vi "Begin.vi"() -> (0 "error out":errorcluster, 1 "CameraDevRef":T5)   [LabVIEW 2011]
doc: "Called before other user functions, this VI is expected to open initial I/O refnums, load in file data, and do all program initialization. Notice that the <B>error out</B> terminal is simply used for data flow. Wiring it to other structures or subVIs ensures that this VI runs first."
uses:
  <vilib>/Rock Robotics/WPI/Camera/WPI_CameraDevRef.ctl
  <vilib>/Rock Robotics/WPI/Encoder/WPI_EncoderDevRef.ctl
  <vilib>/Rock Robotics/SystemInterfaces/Encoder/FPGA_EncoderIdx.ctl
  <vilib>/Rock Robotics/SystemInterfaces/Counter/FPGA_CounterCtrSystemIndex.ctl
  <vilib>/Rock Robotics/WPI/Encoder/WPI_EncoderType.ctl
  <vilib>/Rock Robotics/SystemInterfaces/DIO/FPGA_DIOPWMChannel.ctl
  <vilib>/Rock Robotics/WPI/Joystick/WPI_JoystickDeviceEnum.ctl
  <vilib>/Rock Robotics/WPI/Relay/WPI_RelayDirection.ctl
  <vilib>/Rock Robotics/SystemInterfaces/DIO/FPGA_DIORelayChannel.ctl
  <vilib>/Rock Robotics/SystemInterfaces/Typedef/FPGA_TypedefDigitalModule.ctl
  <vilib>/Rock Robotics/SystemInterfaces/AI/FPGA_AIChannel.ctl
  <vilib>/Rock Robotics/SystemInterfaces/AI/FPGA_AIGyroChannel.ctl
  <vilib>/Rock Robotics/SystemInterfaces/DIO/FPGA_DIOChannel.ctl
  <vilib>/Rock Robotics/WPI/MotorControl/WPI_MotorControlOpen Jaguar.vi
  <vilib>/Rock Robotics/WPI/MotorControl/WPI_MotorControlOpen Victor.vi
  Robot Global Data.vi
  <vilib>/Rock Robotics/WPI/Counter/WPI_CounterDigitalInputToDigitalSource.vi
panel:
  out "EncoderDevRef 2":T1={"DevStatus"={"status"=FALSE, "code"=0, "source"=""}, "EncoderIndex"=enum."Invalid", "CounterIndex"=enum."Invalid", "DistancePerCount"=1.0, "Decoding Type"=enum."4x"}
  out "LDriveEncoder 2":errorcluster
  out "EncoderDevRef":T1={"DevStatus"={"status"=FALSE, "code"=0, "source"=""}, "EncoderIndex"=enum."Invalid", "CounterIndex"=enum."Invalid", "DistancePerCount"=1.0, "Decoding Type"=enum."4x"}
  out "LDriveEncoder":errorcluster
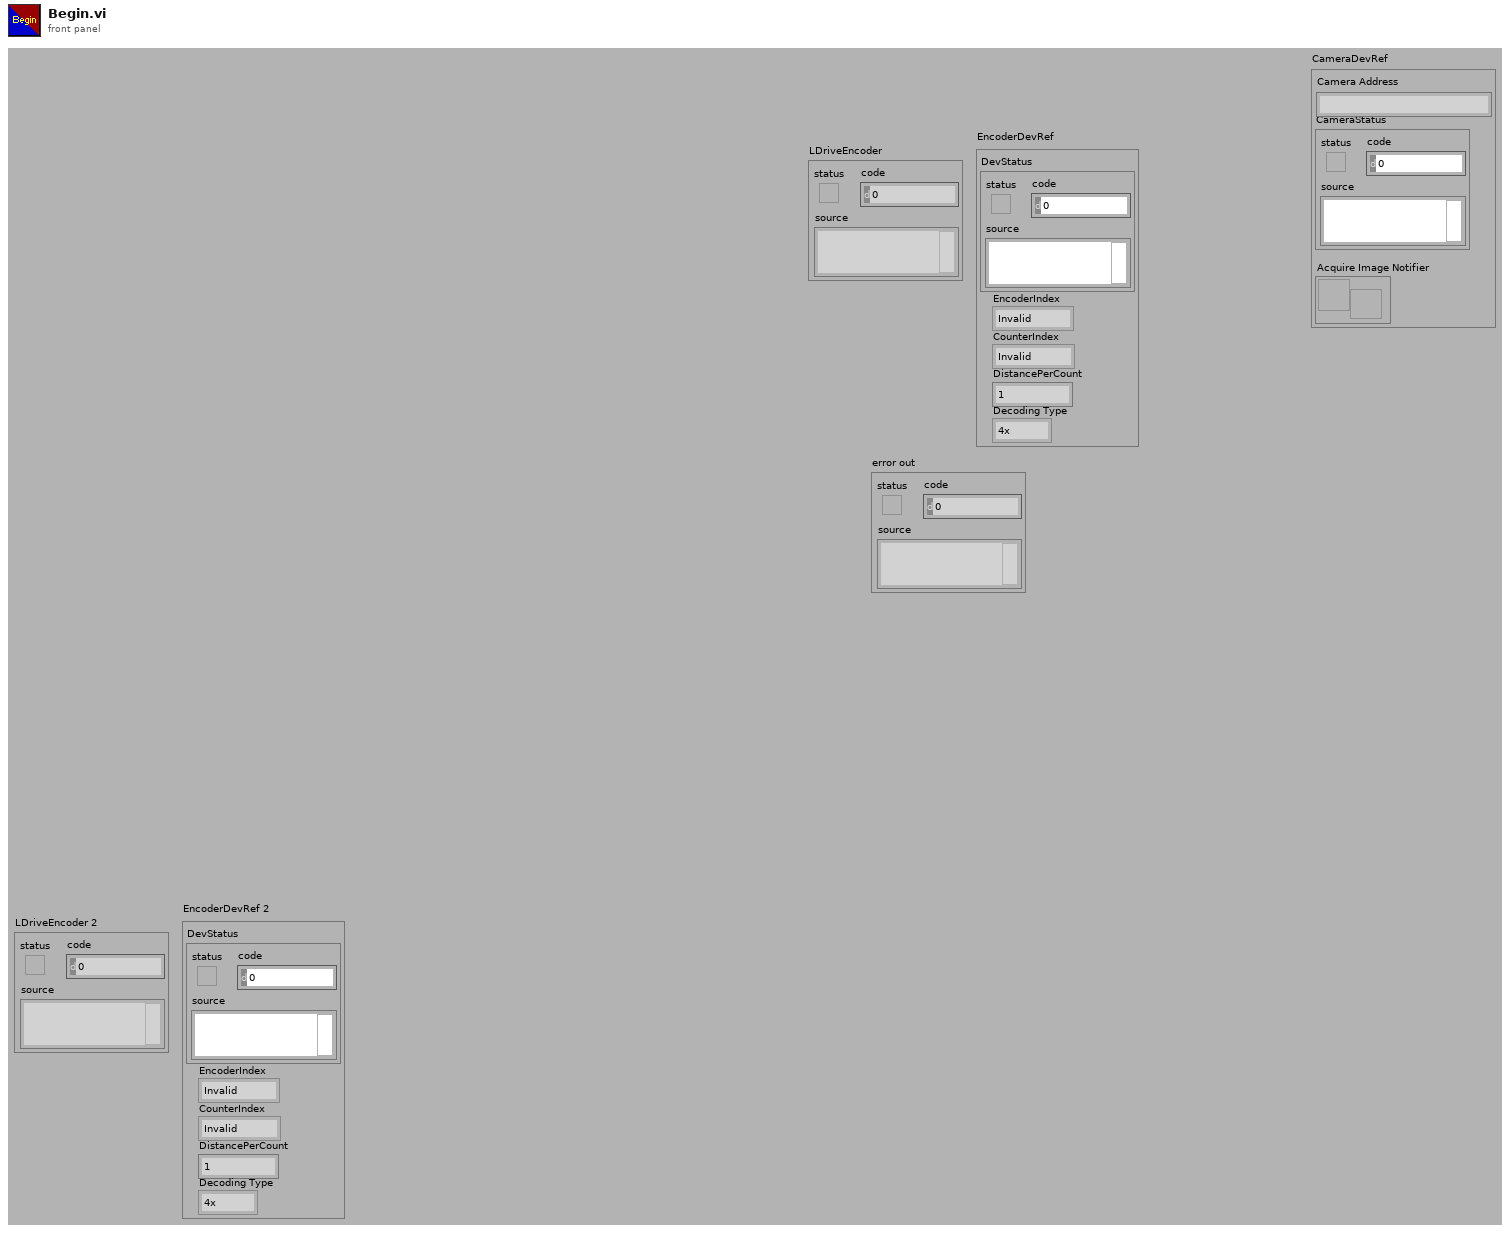
[diagram p1: front panel]
types:
  T1 = typedef "WPI_EncoderDevRef.ctl" = cluster{"DevStatus":errorcluster, "EncoderIndex":T2, "CounterIndex":T3, "DistancePerCount":dbl, "Decoding Type":T4}
  T2 = typedef "FPGA_EncoderIdx.ctl" = enum8{"Enc 0", "Enc 1", "Enc 2", "Enc 3", "Invalid"}
  T3 = typedef "FPGA_CounterCtrSystemIndex.ctl" = enum8{"Ctr 0", "Ctr 1", "Ctr 2", "Ctr 3", "Ctr 4", "Ctr 5", "Ctr 6", "Ctr 7", "Invalid"}
  T4 = typedef "WPI_EncoderType.ctl" = enum16{"1x", "2x", "4x"}
  T5 = typedef "WPI_CameraDevRef.ctl" = cluster{"Camera Address":string, "CameraStatus":errorcluster, "Acquire Image Notifier":refnum<notifier>}
  T6 = typedef "FPGA_DIOChannel.ctl" = enum8{"DIO 1", "DIO 2", "DIO 3", "DIO 4", "DIO 5", "DIO 6", "DIO 7", "DIO 8", "DIO 9", "DIO 10", "DIO 11", "DIO 12", "DIO 13", "DIO 14", "Invalid"}
  T7 = typedef "FPGA_AIGyroChannel.ctl" = enum8{"AI 1", "AI 2", "Invalid"}
  T8 = typedef "FPGA_AIChannel.ctl" = enum8{"AI 1", "AI 2", "AI 3", "AI 4", "AI 5", "AI 6", "AI 7", "AI 8", "Invalid"}
  T9 = typedef "FPGA_TypedefDigitalModule.ctl" = enum16{"Digital Module 1", "Digital Module 2"}
  T10 = typedef "FPGA_DIORelayChannel.ctl" = enum8{"Relay 1", "Relay 2", "Relay 3", "Relay 4", "Relay 5", "Relay 6", "Relay 7", "Relay 8", "Invalid"}
  T11 = typedef "WPI_RelayDirection.ctl" = enum16{"Both directions", "Forward only", "Reverse only"}
  T12 = typedef "WPI_JoystickDeviceEnum.ctl" = enum16{"USB 1", "USB 2", "USB 3", "USB 4", "Kinect 1", "Kinect 2"}
  T13 = typedef "FPGA_DIOPWMChannel.ctl" = enum8{"PWM 1", "PWM 2", "PWM 3", "PWM 4", "PWM 5", "PWM 6", "PWM 7", "PWM 8", "PWM 9", "PWM 10", "Invalid"}
  T14 = typedef "WPI_CameraImageSize.ctl" = enum16{"640x480", "320x240", "160x120"}
  T15 = cluster{"fps":i32, "compression":i32, "Image Size":T14}
  T16 = typedef "WPI_ServoDeviceRef.ctl" = cluster{"DeviceStatus":errorcluster, "Digital Module":T9, "PWM Channel":T13, "DeadBand":T17}
  T17 = typedef "WPI_PWMDeadband.ctl" = cluster{"Name":string, "maxPositivePwm":i32, "minPositivePwm":i32, "centerPwm":i32, "maxNegativePwm":i32, "minNegativePwm":i32, "angularRange":u16}
  T18 = typedef "WPI_MotorControlDeviceRef.ctl" = cluster{"DeviceStatus":errorcluster, "Type":enum16{"PWM", "CAN"}, "PWM":cluster{"Digital Module":T9, "PWM Channel":T13, "DeadBand":T17}, "CAN":cluster{"Device Number":u8, "Control Mode":T19, "Semaphore":T20, "Max Vout":dbl}, "Invert":bool, "TransformRef":T21, "InvTransformRef":T21}
  T19 = typedef "WPI_CANJaguar_ControlMode.ctl" = enum8{"Percent VBus", "Current", "Speed", "Position", "Voltage"}
  T20 = typedef "Semaphore RefNum" = refnum<k1>
  T21 = typedef "WPI_PWMTransform_ConPane.ctl" = refnum<vi>
  T22 = typedef "WPI_DigitalInputDevRef.ctl" = cluster{"DevStatus":errorcluster, "DIO Channel":T6, "Digital Module":T9}
  T23 = typedef "FPGA_CounterEncoderSourceConvertionLVSourceType.ctl" = cluster{"DevStatus":errorcluster, "AnalogTriggerMode?":bool, "DigitalMode":cluster{"Digital Module":T9, "DIO Channel":T24}, "AnalogTriggerMode":cluster{"AnalogTriggerIndex":T25, "OutputType":T26}}
  T24 = typedef "FPGA_DIODigitalSourceChannel.ctl" = enum8{"DIO 1", "DIO 2", "DIO 3", "DIO 4", "DIO 5", "DIO 6", "DIO 7", "DIO 8", "DIO 9", "DIO 10", "DIO 11", "DIO 12", "DIO 13", "DIO 14", "Disabled"}
  T25 = typedef "FPGA_AnalogTriggerIndex.ctl" = enum8{"Trig 0", "Trig 1", "Trig 2", "Trig 3", "Trig 4", "Trig 5", "Trig 6", "Trig 7", "Invalid"}
  T26 = typedef "FPGA_AnalogTriggerOutType.ctl" = enum16{"InWindow", "TriggerState", "Rising", "Falling"}
  T27 = typedef "WPI_CameraWhite Balance Values.ctl" = enum16{"Auto", "Fixed indoor", "Fixed outdoor 1", "Fixed outdoor 2", "Fixed fluorescent 1", "Fixed fluorescent 2", "Hold current"}
  T28 = typedef "WPI_CameraExposure Values.ctl" = enum16{"Auto", "Flicker-free 50 Hz", "Flicker-free 60 Hz", "Hold current"}
  T29 = typedef "WPI_AnalogChannelDevRef.ctl" = cluster{"DevStatus":errorcluster, "Analog Module":T30, "Analog Channel":T8}
  T30 = typedef "FPGA_TypedefAnalogModule.ctl" = enum16{"Analog Module 1", "Analog Module 2"}
  T31 = typedef "WPI_JoystickDevRef.ctl" = cluster{"Device":T12}
  T32 = typedef "WPI_GyroDevRef.ctl" = cluster{"DevStatus":errorcluster, "Analog Module":T30, "Analog Channel":T8, "Offset":dbl, "Gain (VoltsPerDegree/Second)":dbl}
  T33 = typedef "WPI_RelayDevRef.ctl" = cluster{"DevStatus":errorcluster, "Relay Channel":T10, "Digital Module":T9, "Relay Direction":T11}
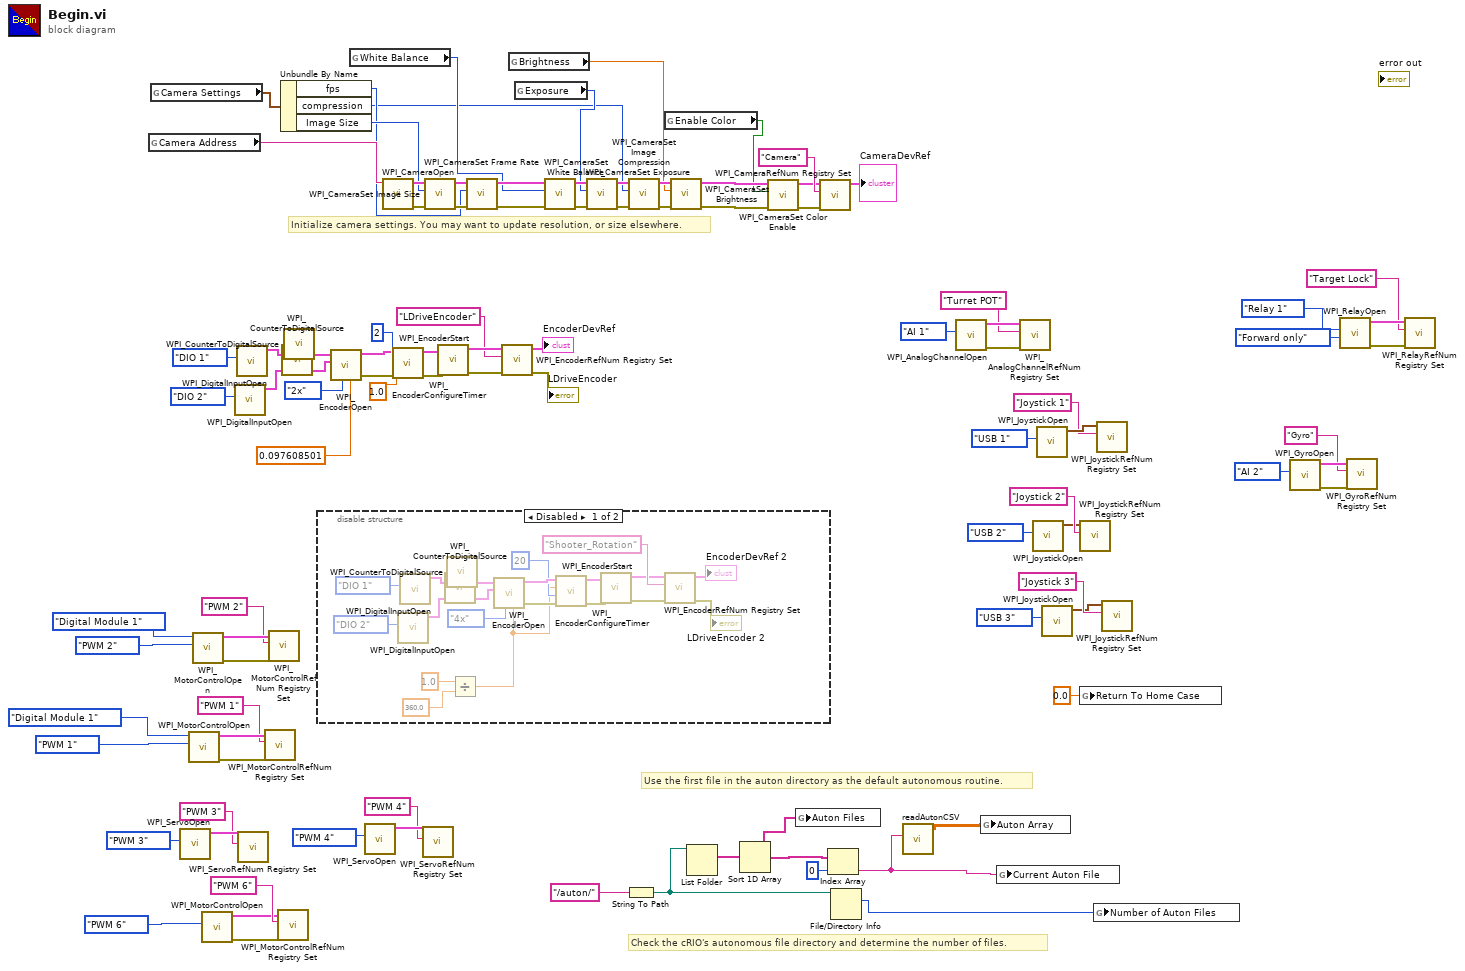
[diagram p0: block diagram]
diagram:
  # "Check the cRIO's autonomous file directory and determine the number of files."
  # "Use the first file in the auton directory as the default autonomous routine."
  # "Initialize camera settings. You may want to update resolution, or size elsewhere."
  n1 = global read "Robot Global Data.vi" "Camera Address"() -> (w84:string)
  n2 = global read "Robot Global Data.vi" "Camera Settings"() -> (w56:T15)
  n3 = call <vilib>:"WPI_ServoOpen.vi"("PWM Channel"=FPGA_DIOPWMChannel."PWM 3") -> ("ServoDeviceRef"=w70:T16)  [unwired: 9 in, 1 out]
  n4 = call-poly <vilib>:"WPI_MotorControlOpen.vi"("PWM Channel"=FPGA_DIOPWMChannel."PWM 1", "Digital Module (Module 1)"=FPGA_TypedefDigitalModule."Digital Module 1") -> ("error out"=w76:errorcluster, "MotorControlDeviceRef"=w79:T18)  [unwired: 8 in]
  n5 = call-poly <vilib>:"WPI_MotorControlOpen.vi"("PWM Channel"=FPGA_DIOPWMChannel."PWM 2", "Digital Module (Module 1)"=FPGA_TypedefDigitalModule."Digital Module 1") -> ("error out"=w77:errorcluster, "MotorControlDeviceRef"=w82:T18)  [unwired: 8 in]
  n6 = call-poly <vilib>:"WPI_MotorControlOpen.vi"("PWM Channel"=FPGA_DIOPWMChannel."PWM 6") -> ("error out"=w65:errorcluster, "MotorControlDeviceRef"=w63:T18)  [unwired: 9 in]
  n7 = call <vilib>:"WPI_DigitalInputOpen.vi"("DIO Channel"=FPGA_DIOChannel."DIO 2") -> ("DigitalInputDevRef"=w5:T22)  [unwired: 9 in, 1 out]
  n8 = call <vilib>:"WPI_DigitalInputOpen.vi"("DIO Channel"=FPGA_DIOChannel."DIO 1") -> ("DigitalInputDevRef"=w2:T22)  [unwired: 9 in, 1 out]
  n9 = call <vilib>:"WPI_ServoRefNum Registry Set.vi"("refnum name"="PWM 3", "ServoDeviceRef"=w70) -> ()  [unwired: 8 in, 2 out]
  n10 = call <vilib>:"WPI_MotorControlRefNum Registry Set.vi"("error in (no error)"=w76, "refnum name"="PWM 1", "MotorControlDevRef"=w79) -> ()  [unwired: 7 in, 2 out]
  n11 = call <vilib>:"WPI_MotorControlRefNum Registry Set.vi"("error in (no error)"=w77, "refnum name"="PWM 2", "MotorControlDevRef"=w82) -> ()  [unwired: 7 in, 2 out]
  n12 = call <vilib>:"WPI_MotorControlRefNum Registry Set.vi"("error in (no error)"=w65, "refnum name"="PWM 6", "MotorControlDevRef"=w63) -> ()  [unwired: 7 in, 2 out]
  n13 = Unbundle By Name(w56) -> ("fps"=w54:i32, "compression"=w51:i32, "Image Size"=w55:T14)
  n14 = call-poly <vilib>:"WPI_CounterToDigitalSource.vi"("DigitalInputDevRef"=w5) -> ("Digital Source"=w6:T23)  [unwired: 6 in]
  n15 = call-poly <vilib>:"WPI_CounterToDigitalSource.vi"("DigitalInputDevRef"=w2) -> ("Digital Source"=w1:T23)  [unwired: 6 in]
  n16 = disable-structure shown="Disabled" {
    frame Disabled {
      n17 = call <vilib>:"WPI_DigitalInputOpen.vi"("DIO Channel"=FPGA_DIOChannel."DIO 2") -> ("DigitalInputDevRef"=w113:T22)  [unwired: 9 in, 1 out]
      n18 = call <vilib>:"WPI_DigitalInputOpen.vi"("DIO Channel"=FPGA_DIOChannel."DIO 1") -> ("DigitalInputDevRef"=w116:T22)  [unwired: 9 in, 1 out]
      n19 = call-poly <vilib>:"WPI_CounterToDigitalSource.vi"("DigitalInputDevRef"=w113) -> ("Digital Source"=w112:T23)  [unwired: 6 in]
      n20 = call-poly <vilib>:"WPI_CounterToDigitalSource.vi"("DigitalInputDevRef"=w116) -> ("Digital Source"=w117:T23)  [unwired: 6 in]
      n21 = Divide(x=1.0, y=360.0) -> (x/y=w98:dbl)
      n22 = call <vilib>:"WPI_EncoderOpen.vi"("DistancePerCount"=w98, "Decoding Type"=WPI_EncoderType."4x", "BSource"=w112, "ASource"=w117) -> ("error out"=w109:errorcluster, "EncoderDevRef"=w108:T1)  [unwired: 6 in]
      n23 = call <vilib>:"WPI_EncoderConfigureTimer.vi"("error in (no error)"=w109, "Number Samples to Average"=u8 20, "Minimum Rate"=w98, "EncoderDevRef"=w108) -> ("error out"=w105:errorcluster, "EncoderDevRef"=w106:T1)  [unwired: 6 in]
      n24 = call <vilib>:"WPI_EncoderStart.vi"("error in (no error)"=w105, "EncoderDevRef"=w106) -> ("error out"=w103:errorcluster, "EncoderDevRef"=w104:T1)  [unwired: 8 in]
      n25 = call <vilib>:"WPI_EncoderRefNum Registry Set.vi"("error in (no error)"=w103, "refnum name"="Shooter_Rotation", "EncoderDevRef"=w104) -> ("error out"=→"LDriveEncoder 2":errorcluster, "EncoderDevRef"=→"EncoderDevRef 2":T1)  [unwired: 7 in]
    }
    frame Enabled {
    }
  }
  n26 = call <vilib>:"WPI_EncoderOpen.vi"("DistancePerCount"=0.097608501, "Decoding Type"=WPI_EncoderType."2x", "BSource"=w6, "ASource"=w1) -> ("error out"=w10:errorcluster, "EncoderDevRef"=w11:T1)  [unwired: 6 in]
  n27 = global read "Robot Global Data.vi" "White Balance"() -> (w53:T27)
  n28 = call <vilib>:"WPI_ServoOpen.vi"("PWM Channel"=FPGA_DIOPWMChannel."PWM 4") -> ("ServoDeviceRef"=w68:T16)  [unwired: 9 in, 1 out]
  n29 = call <vilib>:"WPI_CameraOpen.vi"("Camera Address"=w84) -> ("error out"=w90:errorcluster, "CameraDevRef"=w91:T5)  [unwired: 1 in, 8 out]
  n30 = call <vilib>:"WPI_EncoderConfigureTimer.vi"("error in (no error)"=w10, "Number Samples to Average"=u8 2, "Minimum Rate"=1.0, "EncoderDevRef"=w11) -> ("error out"=w15:errorcluster, "EncoderDevRef"=w14:T1)  [unwired: 6 in]
  n31 = call <vilib>:"WPI_ServoRefNum Registry Set.vi"("refnum name"="PWM 4", "ServoDeviceRef"=w68) -> ()  [unwired: 8 in, 2 out]
  n32 = call <vilib>:"WPI_CameraSet Image Size.vi"("error in (no error)"=w90, "Image Size"=w55, "CameraDevRef"=w91) -> ("error out"=w89:errorcluster, "CameraDevRef Out"=w92:T5)  [unwired: 7 out]
  n33 = call <vilib>:"WPI_EncoderStart.vi"("error in (no error)"=w15, "EncoderDevRef"=w14) -> ("error out"=w17:errorcluster, "EncoderDevRef"=w16:T1)  [unwired: 8 in]
  n34 = call <vilib>:"WPI_CameraSet Frame Rate.vi"("error in (no error)"=w89, "Frame Rate (fps)"=w54, "CameraDevRef"=w92) -> ("error out"=w88:errorcluster, "CameraDevRef Out"=w94:T5)  [unwired: 7 out]
  n35 = call <vilib>:"WPI_EncoderRefNum Registry Set.vi"("error in (no error)"=w17, "refnum name"="LDriveEncoder", "EncoderDevRef"=w16) -> ("error out"=→"LDriveEncoder":errorcluster, "EncoderDevRef"=→"EncoderDevRef":T1)  [unwired: 7 in]
  n36 = global read "Robot Global Data.vi" "Brightness"() -> (w50:dbl)
  n37 = global read "Robot Global Data.vi" "Exposure"() -> (w52:T28)
  n38 = call <vilib>:"WPI_CameraSet White Balance.vi"("error in (no error)"=w88, "White Balance"=w53, "CameraDevRef"=w94) -> ("error out"=w87:errorcluster, "CameraDevRef Out"=w93:T5)  [unwired: 7 out]
  n39 = call <vilib>:"WPI_CameraSet Exposure.vi"("error in (no error)"=w87, "Exposure"=w52, "CameraDevRef"=w93) -> ("error out"=w86:errorcluster, "CameraDevRef Out"=w96:T5)  [unwired: 7 out]
  n40 = String To Path(string="/auton/") -> (path=w31:path)
  n41 = call <vilib>:"WPI_CameraSet Image Compression.vi"("error in (no error)"=w86, "Compression"=w51, "CameraDevRef"=w96) -> ("error out"=w85:errorcluster, "CameraDevRef Out"=w95:T5)  [unwired: 7 out]
  n42 = global read "Robot Global Data.vi" "Enable Color"() -> (w45:bool)
  n43 = call <vilib>:"WPI_CameraSet Brightness.vi"("error in (no error)"=w85, "Brightness"=w50, "CameraDevRef"=w95) -> ("error out"=w48:errorcluster, "CameraDevRef Out"=w49:T5)  [unwired: 7 out]
  n44 = List Folder(path=w31) -> (filenames=w30:string[])  [unwired: 1 in, 5 out]
  n45 = Sort 1D Array(array=w30) -> (sorted array=w25:string[])
  n46 = call <vilib>:"WPI_CameraSet Color Enable.vi"("error in (no error)"=w48, "Color Enabled"=w45, "CameraDevRef"=w49) -> ("error out"=w46:errorcluster, "CameraDevRef Out"=w47:T5)  [unwired: 7 in]
  n47 = global write "Robot Global Data.vi" "Auton Files"(w25) -> ()
  n48 = call <vilib>:"WPI_CameraRefNum Registry Set.vi"("error in (no error)"=w46, "refnum name"="Camera", "CameraDevRef"=w47) -> ("CameraDevRef"=→"CameraDevRef":T5)  [unwired: 8 out]
  n49 = Index Array(array=w25, index=0) -> (element=w27:string)
  n50 = File/Directory Info(path=w31) -> (size=w28:i64)  [unwired: 1 in, 6 out]
  n51 = call "readAutonCSV.vi"("AutonFile"=w27) -> ("AutonArray"=w26:dbl[][])  [unwired: 7 in]
  n52 = call <vilib>:"WPI_AnalogChannelOpen.vi"("Analog Channel"=FPGA_AIChannel."AI 1") -> ("error out"=w35:errorcluster, "AIDeviceRef"=w36:T29)  [unwired: 9 in]
  n53 = global write "Robot Global Data.vi" "Auton Array"(w26) -> ()
  n54 = global write "Robot Global Data.vi" "Current Auton File"(w27) -> ()
  n55 = call <vilib>:"WPI_AnalogChannelRefNum Registry Set.vi"("error in (no error)"=w35, "refnum name"="Turret POT", "AIDeviceRef"=w36) -> ()  [unwired: 7 in, 2 out]
  n56 = call <vilib>:"WPI_JoystickOpen.vi"("JoystickDevice"=WPI_JoystickDeviceEnum."USB 2") -> ("JoystickDevRef"=w72:T31)  [unwired: 10 in]
  n57 = call <vilib>:"WPI_JoystickOpen.vi"("JoystickDevice"=WPI_JoystickDeviceEnum."USB 1") -> ("JoystickDevRef"=w75:T31)  [unwired: 10 in]
  n58 = call <vilib>:"WPI_JoystickOpen.vi"("JoystickDevice"=WPI_JoystickDeviceEnum."USB 3") -> ("JoystickDevRef"=w60:T31)  [unwired: 10 in]
  n59 = call <vilib>:"WPI_JoystickRefNum Registry Set.vi"("refnum name"="Joystick 2", "JoystickDevRef"=w72) -> ()  [unwired: 8 in, 2 out]
  n60 = global write "Robot Global Data.vi" "Return To Home Case"(0.0 ("Return To Home Case")) -> ()
  n61 = global write "Robot Global Data.vi" "Number of Auton Files"(w28) -> ()
  n62 = call <vilib>:"WPI_JoystickRefNum Registry Set.vi"("refnum name"="Joystick 1", "JoystickDevRef"=w75) -> ()  [unwired: 8 in, 2 out]
  n63 = call <vilib>:"WPI_JoystickRefNum Registry Set.vi"("refnum name"="Joystick 3", "JoystickDevRef"=w60) -> ()  [unwired: 8 in, 2 out]
  n64 = call <vilib>:"WPI_GyroOpen.vi"("Analog Channel"=FPGA_AIGyroChannel."AI 2") -> ("error out"=w24:errorcluster, "GyroDevRef"=w23:T32)  [unwired: 8 in, 1 out]
  n65 = call <vilib>:"WPI_RelayOpen.vi"("Relay Direction"=WPI_RelayDirection."Forward only", "Relay Channel"=FPGA_DIORelayChannel."Relay 1") -> ("error out"=w42:errorcluster, "RelayDevRef"=w43:T33)  [unwired: 8 in]
  n66 = call <vilib>:"WPI_GyroRefNum Registry Set.vi"("error in (no error)"=w24, "refnum name"="Gyro", "GyroDevRef"=w23) -> ()  [unwired: 7 in, 2 out]
  n67 = call <vilib>:"WPI_RelayRefNum Registry Set.vi"("error in (no error)"=w42, "refnum name"="Target Lock", "RelayDevRef"=w43) -> ()  [unwired: 7 in, 2 out]
